vi "FRCts20_Backend_TeamRoot_GET_reform.vi"(8 "error in (no error)":errorcluster, 10 "eventdata":variant[][](array[variant]), 11 "recordset data":variant[][](array[variant])) -> (0 "error out":errorcluster, 3 "data string":string)   [LabVIEW 2013, in "FRCts20_Backend_Engine.lvlib"]
doc: "Reforms and returns the list of teams' data"
uses:
  FRCts20_Backend_Engine.lvlib
  FRCts20_Backend_DBCluster_TeamRoot_GET.ctl
  FRCts20_Backend_API/FRCts20_Backend_API_SW.ctl
  FRCts20_Backend_API/FRCts20_Backend_API_TeamRoot.ctl
  <vilib>/addons/database/_DB Variant To Data/Database Variant To Data.xnode
  FRCts20_Backend_API/FRCts20_Backend_API.lvlib
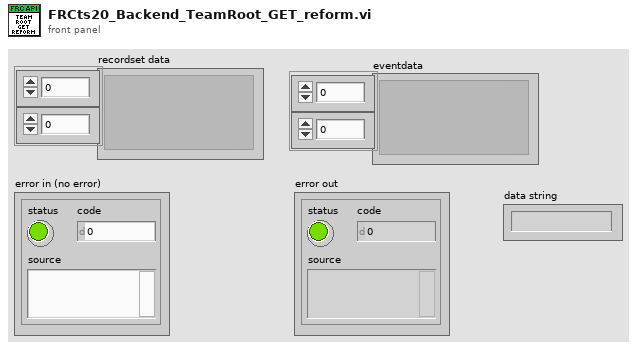
[diagram p1: front panel]
types:
  T1 = typedef "FRCts20_Backend_API.lvlib/FRCts20_Backend_API_TeamRoot.ctl" = cluster{"Teams":cluster{"Team Index":u32, "Team Number":u32, "Team Name":string, "Short Team Name":string, "Nick Name":string, "Robot Name":string, "City":string, "State":string, "Country":string, "Rookie Year":u32, "SWType":T2, "CAN":bool, "Vision":bool, "Kinect":bool, "Tags":string, "Avatar":string, "Events":cluster{"EventIndex":u32, "EventName":string, "IsLive":bool}[]}[], "APIReturn":string}
  T2 = typedef "FRCts20_Backend_API.lvlib/FRCts20_Backend_API_SW.ctl" = string
  T3 = cluster{"TeamIndex":u32, "EventIndex":u32, "EventName":string, "IsLive":bool}[]
  T4 = typedef "FRCts20_Backend_Engine.lvlib/FRCts20_Backend_DBCluster_TeamRoot_GET.ctl" = cluster{"TeamIndex":u32, "TeamNumber":u32, "TeamName":string, "ShortTeamName":string, "NickName":string, "RobotName":string, "City":string, "State":string, "Country":string, "Rookie Year":u32, "SWType":T2, "CAN":bool, "Vision":bool, "Kinect":bool, "Tags":string, "Avatar":string}
  T5 = cluster{"Team Index":u32, "Team Number":u32, "Team Name":string, "Short Team Name":string, "Nick Name":string, "Robot Name":string, "City":string, "State":string, "Country":string, "Rookie Year":u32, "SWType":T2, "CAN":bool, "Vision":bool, "Kinect":bool, "Tags":string, "Avatar":string, "Events":cluster{"EventIndex":u32, "EventName":string, "IsLive":bool}[]}[]
  T6 = cluster{"Team Index":u32, "Team Number":u32, "Team Name":string, "Short Team Name":string, "Nick Name":string, "Robot Name":string, "City":string, "State":string, "Country":string, "Rookie Year":u32, "SWType":T2, "CAN":bool, "Vision":bool, "Kinect":bool, "Tags":string, "Avatar":string, "Events":cluster{"EventIndex":u32, "EventName":string, "IsLive":bool}[]}
  T7 = cluster{"EventIndex":u32, "EventName":string, "IsLive":bool}[]
  T8 = cluster{"EventIndex":u32, "EventName":string, "IsLive":bool}
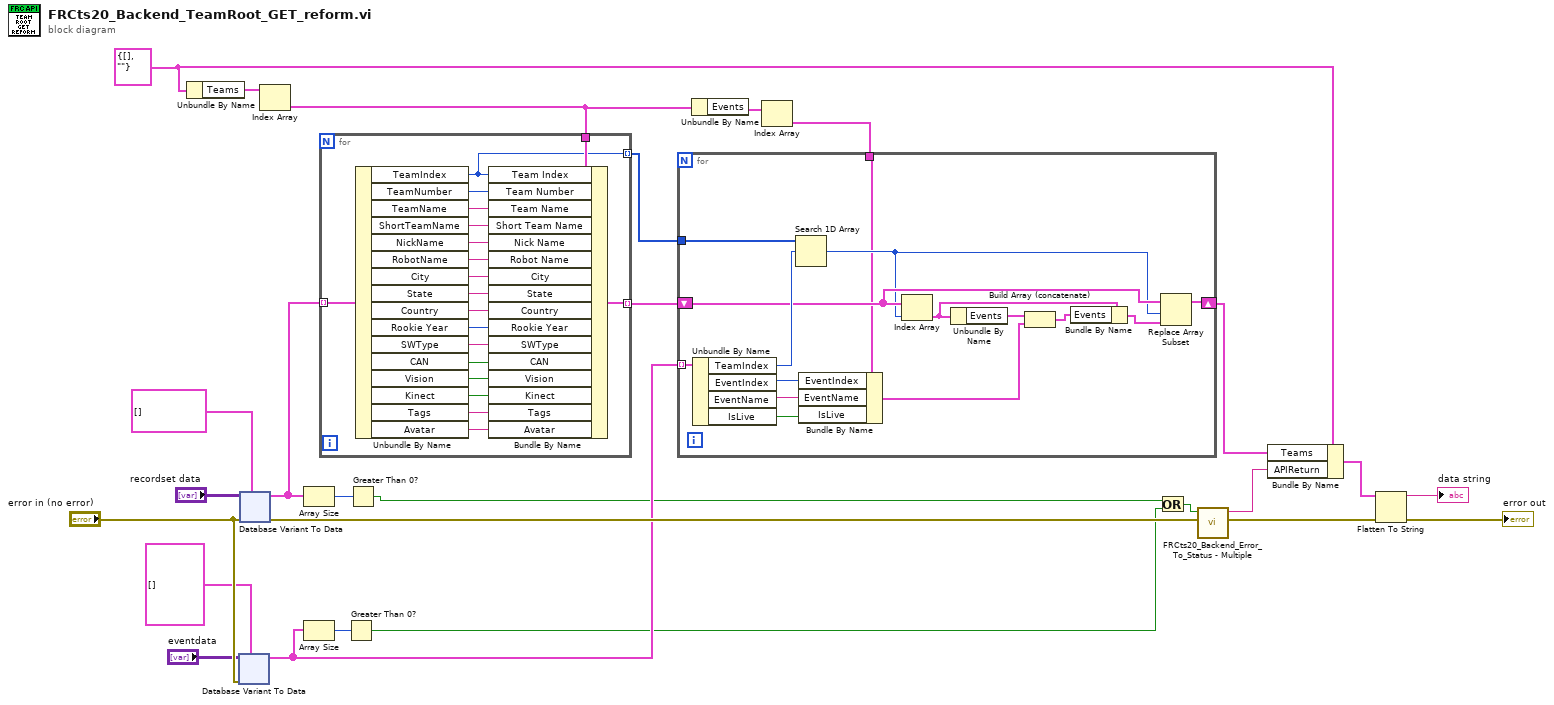
[diagram p0: block diagram]
diagram:
  w12 = T1 {"Teams"=[], "APIReturn"=""} ("Team Root")
  n1 = Unbundle By Name(w12) -> ("Teams"=w17:T5)
  n2 = xnode "Database Variant To Data"("database variant"="eventdata", "error in (no error)"="error in (no error)", "type"=T3 [] ("Events Attending")) -> ("data"=w5:T3)  [unwired: 1 out]
  n3 = xnode "Database Variant To Data"("database variant"="recordset data", "error in (no error)"="error in (no error)", "type"=T4[] []) -> ("data"=w24:T4[], "error out"=w22:errorcluster)
  n4 = Index Array(array=w17) -> (element=w14:T6)  [unwired: 1 in]
  n5 = Array Size(array=w24) -> (size(s)=w6:i32)
  n6 = Array Size(array=w5) -> (size(s)=w4:i32)
  n7 = for {
    tunnel: w24 -> [w45] mode=indexing
    tunnel: w14 -> [w44]
    tunnel: [w31] -> w11 mode=indexing
    tunnel: [w27] -> w10 mode=indexing
    n8 = Unbundle By Name(w45) -> ("TeamIndex"=w27:u32, "TeamNumber"=w43:u32, "TeamName"=w42:string, "ShortTeamName"=w41:string, "NickName"=w40:string, "RobotName"=w39:string, "City"=w38:string, "State"=w37:string, "Country"=w36:string, "Rookie Year"=w35:u32, "SWType"=w34:T2, "CAN"=w30:bool, "Vision"=w29:bool, "Kinect"=w28:bool, "Tags"=w33:string, "Avatar"=w32:string)
    n9 = Bundle By Name(cluster=w44, "Team Index"=w27, "Team Number"=w43, "Team Name"=w42, "Short Team Name"=w41, "Nick Name"=w40, "Robot Name"=w39, "City"=w38, "State"=w37, "Country"=w36, "Rookie Year"=w35, "SWType"=w34, "CAN"=w30, "Vision"=w29, "Kinect"=w28, "Tags"=w33, "Avatar"=w32) -> (w31:T6)
  }
  n10 = Greater Than 0?(x=w4) -> (x > 0?=w2:bool)
  n11 = Greater Than 0?(x=w6) -> (x > 0?=w1:bool)
  n12 = Unbundle By Name(w14) -> ("Events"=w9:T7)
  n13 = Index Array(array=w9) -> (element=w8:T8)  [unwired: 1 in]
  n14 = for {
    tunnel: w5 -> [w60] mode=indexing
    tunnel: w10 -> [w59]
    tunnel: w8 -> [w55]
    shift-right: [w46] -> w7
    shift-left: w11 -> [w57]
    n15 = Unbundle By Name(w60) -> ("TeamIndex"=w58:u32, "EventIndex"=w54:u32, "EventName"=w53:string, "IsLive"=w52:bool)
    n16 = Search 1D Array(1D array=w59, element=w58) -> (index of element=w56:i32)  [unwired: 1 in]
    n17 = Bundle By Name(cluster=w55, "EventIndex"=w54, "EventName"=w53, "IsLive"=w52) -> (w50:T8)
    n18 = Index Array(array=w57, index=w56) -> (element=w49:T6)
    n19 = Unbundle By Name(w49) -> ("Events"=w51:T7)
    n20 = Build Array (concatenate)(w51, w50) -> (w48:T7)
    n21 = Bundle By Name(cluster=w49, "Events"=w48) -> (w47:T6)
    n22 = Replace Array Subset(array=w57, new element=w47, index=w56) -> (w46:T5)
  }
  n23 = Or(x=w1, y=w2) -> (x .or. y?=w3:bool)
  n24 = call "FRCts20_Backend_Error_To_Status - Multiple.vi"("error in (no error)"=w22, "rows affected?"=w3) -> ("error out"=w23:errorcluster, "String"=w25:string)  [unwired: 8 in]
  n25 = Bundle By Name(cluster=w12, "Teams"=w7, "APIReturn"=w25) -> (w20:T1)
  n26 = Flatten To String(anything=w20, error in (no error)=w23) -> (data string=→"data string":string, error out=→"error out":errorcluster)  [unwired: 2 in, 1 out]
